vi "Method_Const.vi"(4 "Array":bool[](array[boolean]), 5 "A":refnum<class "Abs_Boolean_1D.lvclass">) -> (1 "Result":refnum<class "Abs_Boolean_1D.lvclass">)   [LabVIEW 2021, in "AND_Bool_1D.lvclass"]
uses:
  AND_Bool_1D.lvclass
  Abs_Types/Boolean_1D/Abs_Boolean_1D.lvclass
  C:/TSA/LV_Abstract/Source/Functions/Support/Function/Two Terminal/Bool_1D/AbsFunc_Two Term_Bool_1D.lvclass
  C:/TSA/LV_Abstract/Source/Abs_Types/Boolean_1D/Abs_Boolean_1D.lvclass
  Support/Function/Two Terminal/Bool_1D/AbsFunc_Two Term_Bool_1D.lvclass/AbsFunc_Two Term_Bool_1D.ctl
  Support/Function/Two Terminal/Bool_1D/Properties/Write Bool1D A.vi
  Support/Function/Two Terminal/Bool_1D/Properties/Write Bool1D B.vi
  Constants/Support/Bool_1D/Const_Bool_1D.lvclass
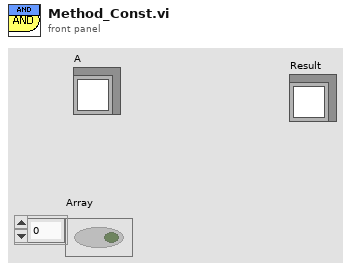
[diagram p1: front panel]
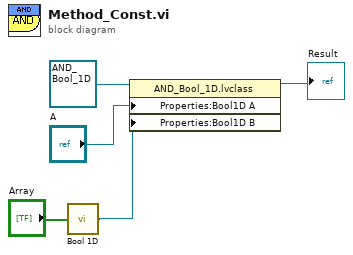
[diagram p0: block diagram]
diagram:
  n1 = call "Bool 1D.vi"("Array"="Array") -> ("Abs_Boolean_1D.lvclass"=w1:refnum<class "Abs_Boolean_1D.lvclass">)  [unwired: 4 in]
  n2 = property class="AND_Bool_1D.lvclass"(reference=refnum<class "AND_Bool_1D.lvclass"> refnum ("Functions.lvlib:Logic.lvlib:AND.lvclass"), "Properties:Bool1D A"="A", "Properties:Bool1D B"=w1) -> (reference out=→"Result":refnum<class "AND_Bool_1D.lvclass">)  [unwired: 1 in, 1 out]
